vi "RunLoadSummary.vi"() -> ()   [LabVIEW 2012]
uses:
  Global1.vi
  <vilib>/Utility/file.llb/Read From Spreadsheet File (string).vi
panel:
  out "error out":errorcluster
  out "Output":string
  out "OK":bool
  out "element":string
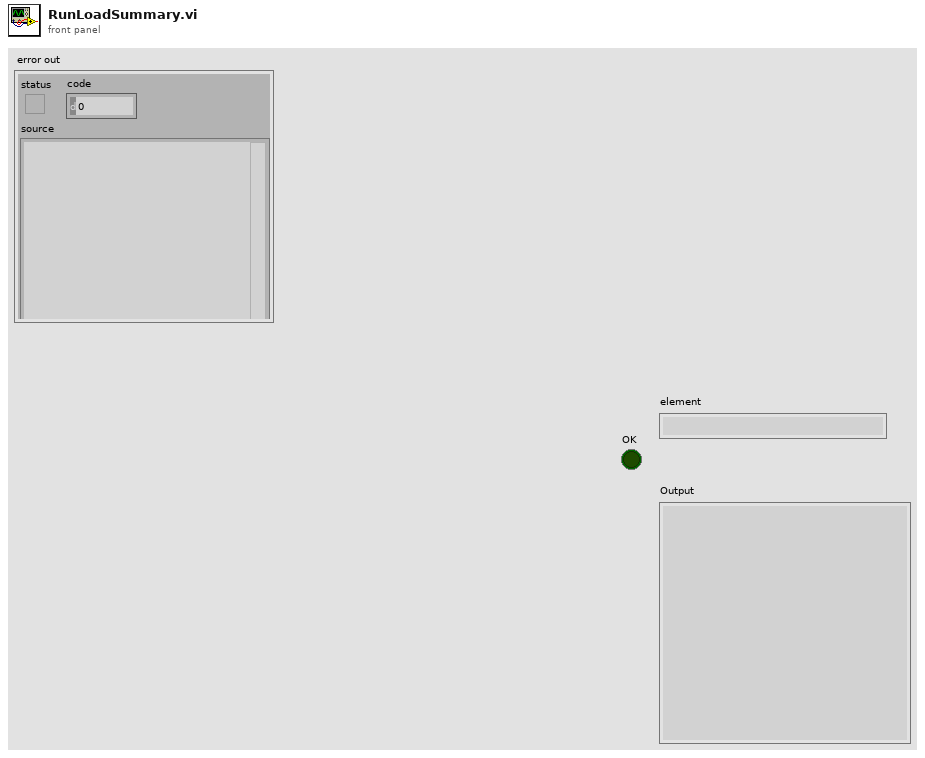
[diagram p1: front panel]
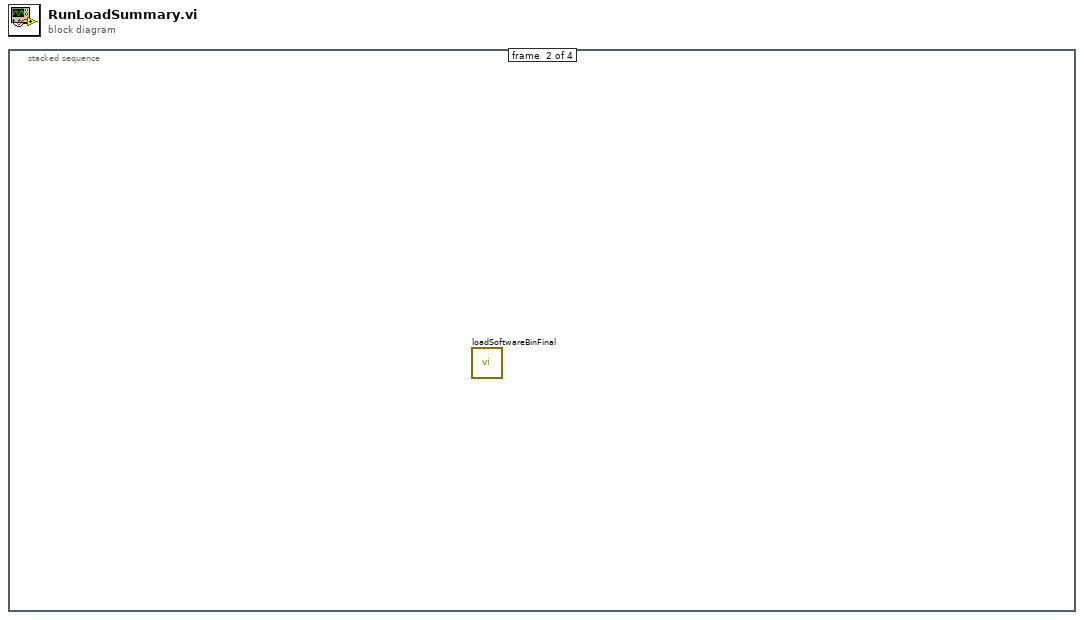
[diagram p0: block diagram]
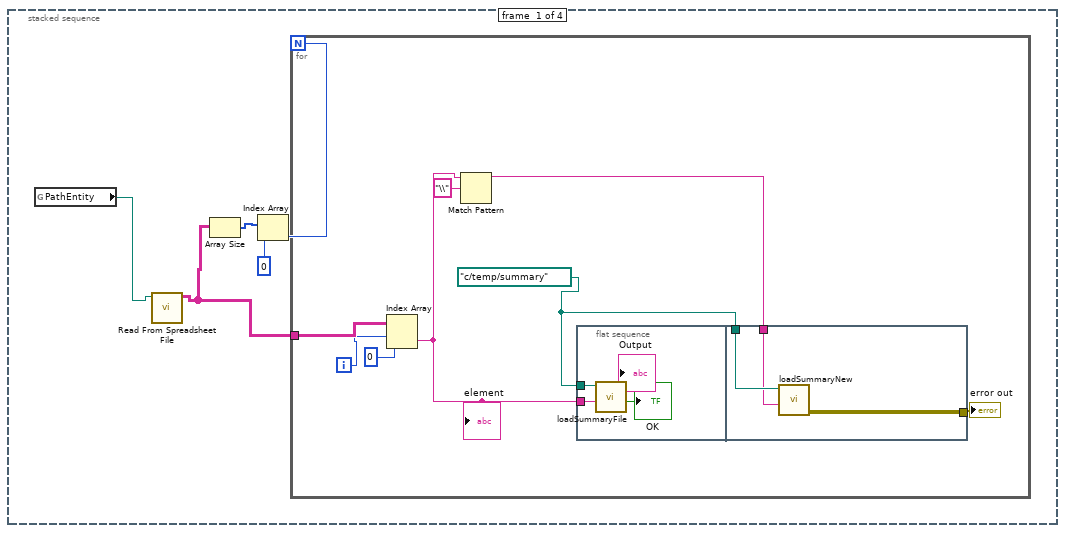
[diagram p2: hidden frame]
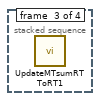
[diagram p3: hidden frame]
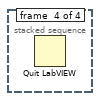
[diagram p4: hidden frame]
diagram:
  n1 = stacked-sequence {
    frame #0 {
      n2 = global read "Global1.vi" "PathEntity"() -> (w1:path)
      n3 = call-poly <vilib>:"Read From Spreadsheet File.vi"("file path (dialog if empty)"=w1) -> ("all rows"=w2:string[][])  [unwired: 6 in, 4 out]
      n4 = Array Size(array=w2) -> (size(s)=w5:i32[])
      n5 = Index Array(array=w5, index=0) -> (element=w3:i32)
      n6 = for {
        N: w3 -> [_]
        tunnel: w2 -> [w13]
        i -> [w11]
        w10 = path "c:/temp/summary" ("working directory")
        n7 = Index Array(array=w13, index (row)=w11, index (col)=0 ("disabled index (col)")) -> (element=w7:string)
        "element" <- w7
        n8 = Match Pattern(string=w7, regular expression="\\") -> (before substring=w6:string)  [unwired: 1 in, 3 out]
        n9 = flat-sequence {
          tunnel: w7 -> [w17]
          tunnel: w10 -> [w16]
          tunnel: w10 -> [w20]
          tunnel: [w19] -> w9
          tunnel: w6 -> [w18]
          frame #0 {
            n10 = call "loadSummaryFile.vi"("folder"=w17, "working directory"=w16) -> ("OK"=→"OK":bool, "Output"=→"Output":string)  [unwired: 8 in]
          }
          frame #1 {
            n11 = call "loadSummaryNew.vi"("machine"=w18, "path"=w20) -> ("error out"=w19:errorcluster)  [unwired: 9 in]
          }
        }
        "error out" <- w9
      }
    }
    frame #1 {
      n12 = call "loadSoftwareBinFinal.vi"() -> ()  [unwired: 12 in]
    }
    frame #2 {
      n13 = call "UpdateMTsumRTToRT1.vi"() -> ()  [unwired: 12 in]
    }
    frame #3 {
      n14 = Quit LabVIEW() -> ()  [unwired: 1 in]
    }
  }
